vi "VtoZ.vi"(1 "Voltage IN":dbl) -> (0 "Zpos OUT (um)":dbl)   [LabVIEW 2015]
panel:
  in  "Calibration method":u16(ring)=1 items=["Theoretical", "Experimental"]
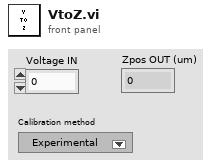
[diagram p1: front panel]
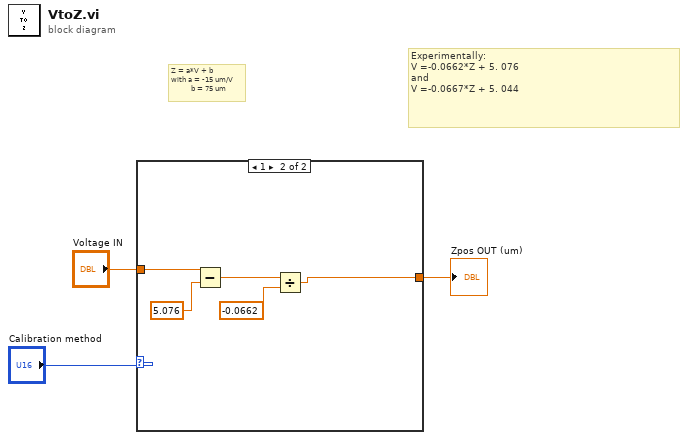
[diagram p0: block diagram]
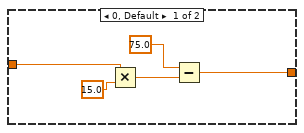
[diagram p2: hidden frame]
diagram:
  # "Experimentally:\nV =-0.0662*Z + 5. 076\nand\nV =-0.0667*Z + 5. 044"
  # "Z = a*V + b\nwith a = -15 um/V\n          b = 75 um"
  n1 = case shown="1" "Calibration method" {
    tunnel: "Voltage IN" -> [w8 w13]
    tunnel: [w4 w10] -> w2
    frame 0, Default {
      n2 = Multiply(x=w8, y=15.0) -> (x*y=w6:dbl)
      n3 = Subtract(x=75.0, y=w6) -> (x-y=w4:dbl)
    }
    frame 1 {
      n4 = Subtract(x=w13, y=5.076) -> (x-y=w11:dbl)
      n5 = Divide(x=w11, y=-0.0662) -> (x/y=w10:dbl)
    }
  }
  "Zpos OUT (um)" <- w2
